vi "Test DRAM Half Size.vi"(7 "fifo depth":T2=23 items=["4"=2, "8"=3, "16"=4, "32"=5, "64"=6, "128"=7, "256"=8, "512"=9, "1024"=10, "2048"=11, "4096"=12, "8192"=13, "16384"=14, "32768"=15, "65536"=16, "131072"=17, "262144"=18, "524288"=19, "1048576"=20, "2097152"=21, "4194304"=22, "8388608"=23, "16777216"=24, "33554432"=25, "67108864"=26, "134217728"=27, "268435456"=28, "536870912"=29, "1073741824"=30, "2147483648"=31, "4294967296"=32], 10 "arbiter configuration":T1={"write grant time (clocks)"=100, "read grant time (clocks)"=100}, 11 "Points to Generate":u32=200000000 format="%.0p") -> (2 "Pass?":bool, 3 "Write Throughput (Bytes/sec)":u32 format="%.2p")   [LabVIEW 2011]
uses:
  <instrlib>/RF-RIO/FIFO/FPGA/Private/FIFO Depth - 32-bit Address.ctl
  <instrlib>/RF-RIO/Memory/FPGA/Interface/Timeslot Arbiter Configuration.ctl
  <vilib>/Platform/TimedLoop/XDataNode/timing_clust.ctl
  <vilib>/Platform/TimedLoop/XDataNode/nitl_modes.ctl
  <vilib>/Platform/TimedLoop/XDataNode/wakeup.ctl
  <vilib>/Platform/TimedLoop/XDataNode/XDataNode.xnode
  <vilib>/Platform/TimedLoop/XDataNode/XDNodeRunTimeDep.lvlib
  <instrlib>/RF-RIO/FIFO/FPGA/FIFO.lvlib
  <instrlib>/RF-RIO/Memory/FPGA/Memory.lvlib
panel:
  out "Read Throughput (Bytes/sec)":u32 format="%.2p"
  out "Gen. Points Done":u32 format="%.0p"
  out "Generation Done?":bool
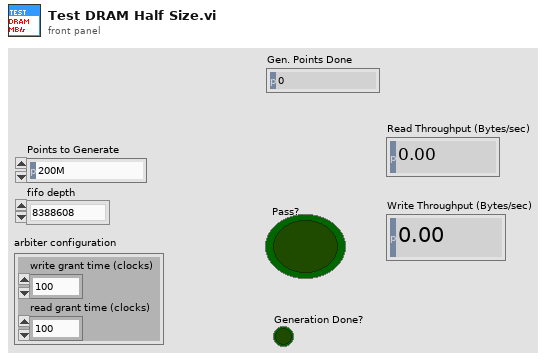
[diagram p1: front panel]
types:
  T1 = typedef "Memory.lvlib/Timeslot Arbiter Configuration.ctl" = cluster{"write grant time (clocks)":u16, "read grant time (clocks)":u16}
  T2 = typedef "FIFO.lvlib/FIFO Depth - 32-bit Address.ctl" = u8
  T3 = typedef "XDNodeRunTimeDep.lvlib/timing_clust.ctl" = cluster{"Expected End [f-1]":u64, "Actual End [f-1]":u64, "Finished Late? [f-1]":bool, "Expected End [i-1]":u64, "Actual End [i-1]":u64, "Finished Late? [i-1]":bool, "Expected Start [i]":u64, "Actual Start [i]":u64, "Expected Start [f]":u64, "Actual Start [f]":u64, "Source Name":string, "Structure Name":string, "Period":i64, "Deadline":i64, "Offset":i64, "Start":i64, "Priority":i32, "Timeout":i32, "Mode":T4, "Wakeup Reason":T5, "Error":errorcluster, "Source Type":string, "Secondary Source Type":string, "Global End Time":u64, "Global Start Time":u64, "Frame Duration":u64, "Iteration Duration":u64, "Assigned CPU":i32, "I/O Scan Engine Mode":u32}
  T4 = typedef "XDNodeRunTimeDep.lvlib/nitl_modes.ctl" = enum32{"No Change", "Process missed periods, maintain original phase", "Discard missed periods, maintain original phase", "Process missed periods, ignore original phase", "Discard missed periods, ignore original phase"}
  T5 = typedef "XDNodeRunTimeDep.lvlib/wakeup.ctl" = enum32{"Normal", "Aborted", "Asynchronous wakeup", "Timing source error", "Timed loop error", "Timeout"}
  T6 = cluster{"fifo1 memory":refnum<k21>, "fifo2 memory":refnum<k21>}
  T7 = typedef "Data Type (256).ctl" = cluster{"Bank0. High":u64, "Bank0. Low":u64, "Bank1. High":u64, "Bank1. Low":u64}
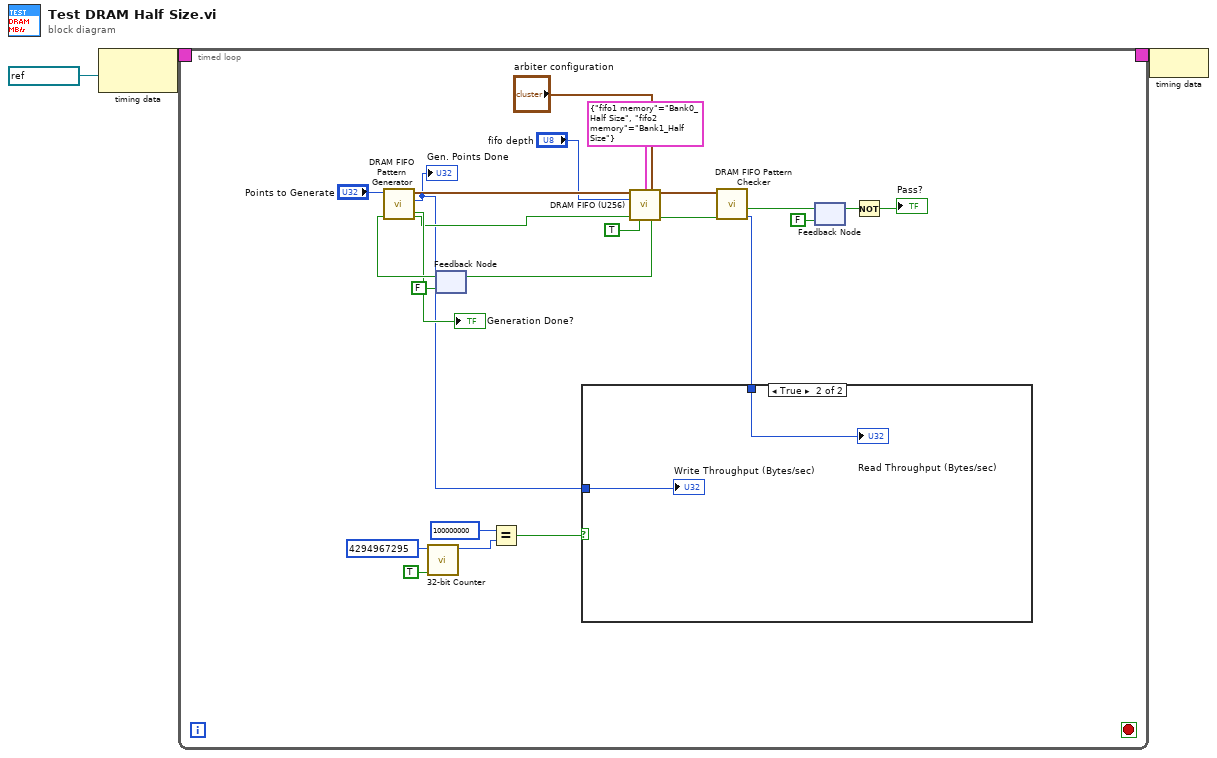
[diagram p0: block diagram]
diagram:
  n1 = node-c288(refnum<k21> "100MHz" ("Source Name")) -> (w3:T3)
  n2 = timed-loop {
    timing: w3 -> [_]
    timing-out: [_] -> w2
    stop <- _ stop-if-true
    n3 = call "32-bit Counter.vi"("INC?"=TRUE, "rollover"=u32 4294967295) -> ("count"=w9:u32)  [unwired: 9 in]
    n4 = feedback #1(FALSE ("Ready for Input")) -> (w24:bool)
    n5 = call "DRAM FIFO Pattern Generator.vi"("Generate Point"=w24, "Points to Generate"="Points to Generate") -> ("Output Valid"=w16:bool, "Generation Done?"=→"Generation Done?":bool, "Points Done"=w5:u32, "Output Data"=w26:T7)  [unwired: 6 in]
    "Gen. Points Done" <- w5
    n6 = Equal?(x=u32 100000000, y=w9) -> (x = y?=w10:bool)
    n7 = call "DRAM FIFO (U256).vi"("Input Data"=w26, "Memory"=T6 {"fifo1 memory"="Bank0_Half Size", "fifo2 memory"="Bank1_Half Size"}, "arbiter configuration"="arbiter configuration", "fifo depth"="fifo depth", "input valid"=w16, "ready for output"=TRUE) -> ("Output Data"=w14:T7, "Ready for Input"=w25:bool, "Output Valid"=w13:bool)  [unwired: 4 in, 3 out]
    n8 = feedback-in #1(w25) -> ()
    n9 = call "DRAM FIFO Pattern Checker.vi"("Input Valid"=w13, "Input Data"=w14) -> ("Points Done"=w4:u32, "Pattern Match Ever Fail?"=w23:bool)  [unwired: 3 in, 5 out]
    n10 = case shown="True" w10 {
      tunnel: w5 -> [_ w29]
      tunnel: w4 -> [_ w28]
      frame False {
      }
      frame True {
        "Write Throughput (Bytes/sec)" <- w29
        "Read Throughput (Bytes/sec)" <- w28
      }
    }
    n11 = feedback #2(FALSE ("Pattern Match Ever Fail?")) -> (w12:bool)
    n12 = feedback-in #2(w23) -> ()
    n13 = Not(x=w12) -> (.not. x?=→"Pass?":bool)
  }
  n14 = node-c288(w2) -> ()
